vi "Cart Pendulum Model.vi"(10 "States In":T1 format="%.4f", 11 "PWM":dbl) -> (3 "States Out":T1 format="%.4f")   [LabVIEW 2018]
uses:
  States.ctl
  <vilib>/Simulation/Implementation/Shared/SIMSCR Execution Mode.ctl
  <vilib>/Simulation/Scripting/Companion Diagram/SimConfigNode/SimParams.ctl
  <vilib>/Simulation/Scripting/Companion Diagram/SimConfigNode/_simSolvers.ctl
  <vilib>/Simulation/Param Hierarchy/Typedefs/SIMPH Param Control Actions.ctl
  <vilib>/Simulation/Implementation/Shared/SIM limit type.ctl
  <vilib>/Simulation/Implementation/Shared/NILVSim_ParamChanged.vi
  <vilib>/Simulation/Implementation/Shared/NILVSIM_BeginStep.vi
  <vilib>/Simulation/ContinuousLinear/Implementation/NILVSim Integrator new.llb/SIM Integrator Distributor (vector).vi
  <vilib>/Simulation/ContinuousLinear/Implementation/NILVSim Integrator new.llb/SIM Integrator Collector (vector).vi
  <vilib>/Simulation/Implementation/Shared/NILVSim_Manager.vi
  <vilib>/Utility/error.llb/Clear Errors.vi
  <vilib>/Simulation/Implementation/Shared/NILVSim_FinalizeModel.vi
  <vilib>/Simulation/Implementation/Shared/SIM Unbundle Sim Info.vi
  <vilib>/Simulation/Implementation/Shared/SIMSH Read Queue.vi
  <vilib>/Simulation/Implementation/Shared/NILVSim_Initialize.vi
  <vilib>/Simulation/Utility/Implementation/NILVSim Get Time and IsAcceptedStep.vi
  <vilib>/Simulation/Implementation/Shared/NILVSim_GetModelError.vi
  <vilib>/Simulation/Implementation/Shared/SIM SimErrorHandler.vi
  <vilib>/Simulation/Implementation/Shared/SIM Bundle Sim Info.vi
  <vilib>/Simulation/Scripting/Companion Diagram/SimConfigNode/SimDog.xnode
  <vilib>/Simulation/Implementation/XNodeFramework/SimXNode/SimX.xnode
  <vilib>/Simulation/ContinuousLinear/Implementation/NILVSim Integrator new.llb/SIM Integrator (vector).vi
  <vilib>/Simulation/Implementation/Shared/NI_SIM_Implementation.lvlib
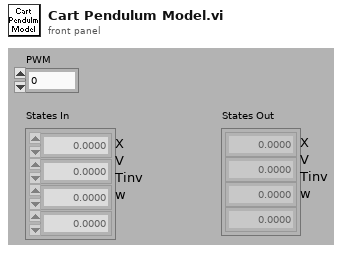
[diagram p1: front panel]
types:
  T1 = typedef "States.ctl" = dbl[]
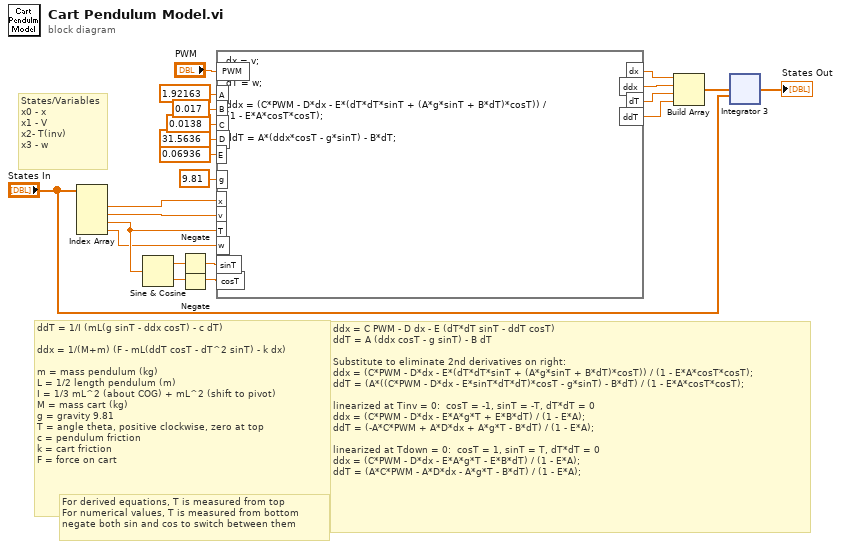
[diagram p0: block diagram]
diagram:
  # "States/Variables\nx0 - x\nx1 - V\nx2- T(inv)\nx3 - w"
  # "ddx = C PWM - D dx - E (dT*dT sinT - ddT cosT)\nddT = A (ddx cosT - g sinT) - B dT\n\nSubstitute to eliminate 2nd derivatives on right:\nddx = (C*PWM - D*dx - E*(dT*dT*sinT + (A*g*sinT + B*dT)*cosT)) / (1 - E*A*cosT*cosT);\nddT = (A*((C*PWM - D*dx - E*sinT*dT*dT)*cosT - g*sinT) - B*dT) / (1 - E*A*cosT*cosT);\n\nlinearized at Tinv = 0:  cosT = -1, sinT = -T, dT*dT = 0\nddx = (C*PWM - D*dx - E*A*g*T + E*B*dT) / (1 - E*A);\nddT = (-A*C*PWM + A*D*dx + A*g*T - B*dT) / (1 - E*A);\n\nlinearized at Tdown = 0:  cosT = 1, sinT = T, dT*dT = 0\nddx = (C*PWM - D*dx - E*A*g*T - E*B*dT) / (1 - E*A);\nddT = (A*C*PWM - A*D*dx - A*g*T - B*dT) / (1 - E*A);"
  # "For derived equations, T is measured from top\nFor numerical values, T is measured from bottom\nnegate both sin and cos to switch between them"
  # "ddT = 1/I (mL(g sinT - ddx cosT) - c dT)\n\nddx = 1/(M+m) (F - mL(ddT cosT - dT^2 sinT) - k dx)\n\nm = mass pendulum (kg)\nL = 1/2 length pendulum (m)\nI = 1/3 mL^2 (about COG) + mL^2 (shift to pivot)\nM = mass cart (kg)\ng = gravity 9.81\nT = angle theta, positive clockwise, zero at top\nc = pendulum friction\nk = cart friction\nF = force on cart"
  n1 = Index Array(array="States In") -> (element #1=w11:dbl, element #2=w10:dbl, element #3=w9:dbl, element #4=w8:dbl)  [unwired: 4 in]
  n2 = Sine & Cosine(0:w9) -> (1:w18:dbl, 2:w17:dbl)
  n3 = Negate(x=w18) -> (-x=w20:dbl)
  n4 = Negate ("Negate 2")(x=w17) -> (-x=w19:dbl)
  n5 = formula code="dx = v;\n\ndT = w;\n\nddx = (C*PWM - D*dx - E*(dT*dT*sinT + (A*g*sinT + B*dT)*cosT)) / \n(1 - E*A*cosT*cosT);\n\nddT = A*(ddx*cosT - g*sinT) - B*dT;"("PWM"="PWM", "x"=w11, "v"=w10, "T"=w9, "w"=w8, "cosT"=w19, "sinT"=w20, "A"=1.92163 ("input variable 3"), "B"=0.017 ("input variable 4"), "C"=0.0138 ("input variable 5"), "D"=31.5636 ("input variable 6"), "E"=0.06936 ("input variable"), "g"=9.81 ("input variable 2")) -> ("dx"=w2:dbl, "ddx"=w7:dbl, "dT"=w3:dbl, "ddT"=w6:dbl)
  n6 = Build Array(w2, w7, w3, w6) -> (w5:dbl[])
  n7 = xnode ("Integrator 3")("input"=w5, "initial condition"="States In") -> ("output"=→"States Out":dbl[])  [unwired: 8 in, 2 out]
